vi "2023 Teleop Arm PID Control.vi"(3 "error in (no error)":errorcluster, 4 "reinitialize? (F)":bool, 5 "Joystick Y Axis":dbl) -> (0 "error out":errorcluster, 1 "Commanded\nSet Output":dbl, 2 "Sensor Position":dbl)   [LabVIEW 2020]
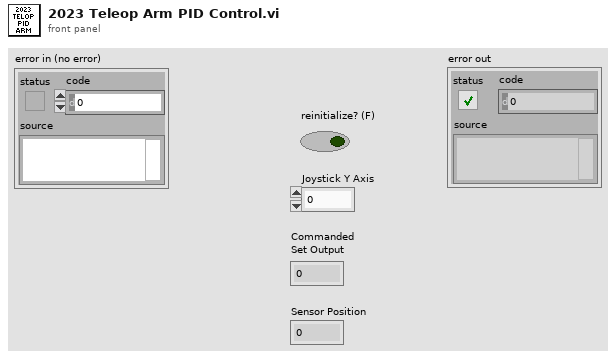
[diagram p1: front panel]
types:
  T1 = typedef "WPI_MotorControlDeviceRef.ctl" = cluster{"DeviceStatus":errorcluster, "Type":T2, "PWM":cluster{"PWM Channel":T3, "DeadBand":T4}, "CAN":cluster{"Device Number":u8, "SetOutput VI Ref":variant, "GetOutput VI Ref":variant, "Enable VI Ref":variant, "Disable VI Ref":variant, "Data":variant}, "Invert":bool, "DIO PWM":cluster{"PWM \"Enable\" Channel":T3, "DIOChannel":T5, "PWM Rate":dbl}}
  T2 = typedef "WPI_MotorControlType.ctl" = enum16{"PWM", "CAN", "DIO PWM"}
  T3 = typedef "FPGA_DIOPWMChannel.ctl" = enum8{"PWM 0", "PWM 1", "PWM 2", "PWM 3", "PWM 4", "PWM 5", "PWM 6", "PWM 7", "PWM 8", "PWM 9", "PWM MXP 0", "PWM MXP 1", "PWM MXP 2", "PWM MXP 3", "PWM MXP 4", "PWM MXP 5", "PWM MXP 6", "PWM MXP 7", "PWM MXP 8", "PWM MXP 9", "Invalid"}
  T4 = typedef "WPI_PWMDeadband.ctl" = cluster{"Name":string, "maxPositivePwm":i32, "minPositivePwm":i32, "centerPwm":i32, "maxNegativePwm":i32, "minNegativePwm":i32, "angularRange":u16}
  T5 = typedef "FPGA_DIOChannel.ctl" = enum8{"DIO 0", "DIO 1", "DIO 2", "DIO 3", "DIO 4", "DIO 5", "DIO 6", "DIO 7", "DIO 8", "DIO 9", "DIO MXP 0", "DIO MXP 1", "DIO MXP 2", "DIO MXP 3", "DIO MXP 4", "DIO MXP 5", "DIO MXP 6", "DIO MXP 7", "DIO MXP 8", "DIO MXP 9", "DIO MXP 10", "DIO MXP 11", "DIO MXP 12", "DIO MXP 13", "DIO MXP 14", "DIO MXP 15", "SPI Port CS1", "SPI Port CS2", "SPI Port CS3", "SPI Port MISO", "SPI Port MOSI", "Invalid"}
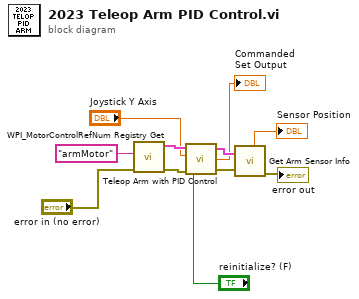
[diagram p0: block diagram]
diagram:
  n1 = call <vilib>:"WPI_MotorControlRefNum Registry Get.vi"("error in (no error)"="error in (no error)", "refnum name"="armMotor") -> ("error out"=w7:errorcluster, "MotorControlDevRef"=w9:T1)  [unwired: 8 in]
  n2 = call "Teleop Arm with PID Control.vi"("error in (no error)"=w7, "reinitialize? (F)"="reinitialize? (F)", "Joystick Command"="Joystick Y Axis", "MotorControlDevRef"=w9) -> ("error out"=w6:errorcluster, "Commanded\nSet Output"=→"Commanded\nSet Output":dbl, "MotorControlOutput"=w5:T1)
  n3 = call "Get Arm Sensor Info.vi"("error in (no error)"=w6, "MotorControlDevRef"=w5) -> ("error out"=→"error out":errorcluster, "Sensor Position"=→"Sensor Position":dbl)  [unwired: 3 out]
